vi "WSVCAP SHL Host TL RFFE Read.vi"(0 "Write Data In [DUT Ordered]":u8[][](array[numeric]) format="%02x", 7 "Socket Mask":u64=1 format="%016x", 11 "error in":errorcluster, 13 "Log (T)":bool=TRUE, 14 "FPGA":T1) -> (4 "Read Data Out":u8[][](array[numeric]) format="%.0x", 15 "error out":errorcluster)   [LabVIEW 2017]
uses:
  Type Defs/WSVCAP SHL FPGA Enum.ctl
  Type Defs/WSVCAP SHL Function Enum.ctl
panel:
  out "Status":u8[](array[numeric])
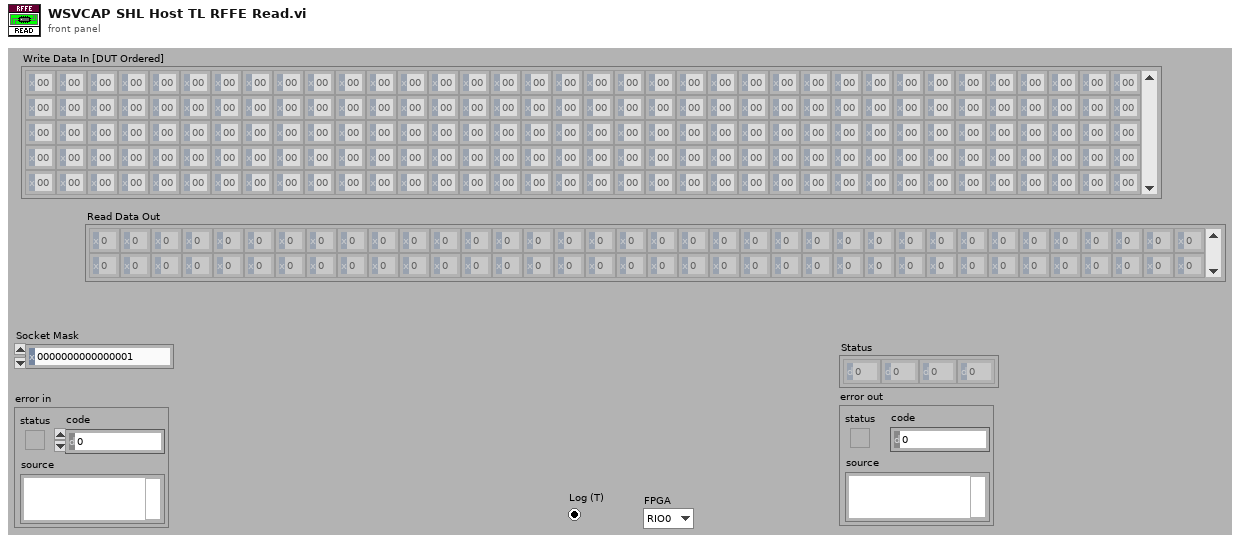
[diagram p1: front panel]
types:
  T1 = typedef "WSVCAP SHL FPGA Enum.ctl" = enum16{"RIO0", "RIO1"}
  T2 = typedef "WSVCAP SHL Function Enum.ctl" = enum16{"Initialize", "Configure I2C", "Configure RFFE", "Write I2C", "Read I2C", "Write RFFE", "Read RFFE", "Start RFFE Cycle", "Stop RFFE Cycle", "Get Status", "Close"}
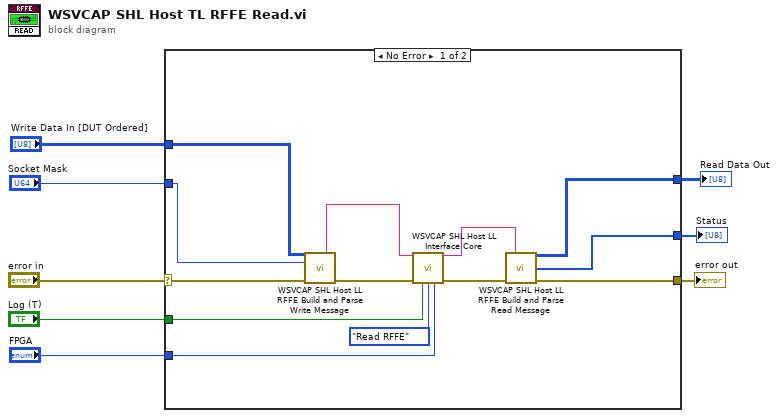
[diagram p0: block diagram]
diagram:
  n1 = case shown="No Error" "error in" {
    selector: "error in" -> [w14 w22]
    tunnel: [w18 w22] -> w8
    tunnel: "Socket Mask" -> [w12 _]
    tunnel: [w17 _] -> w5
    tunnel: [w16 _] -> w4
    tunnel: "Log (T)" -> [w15 _]
    tunnel: "Write Data In [DUT Ordered]" -> [w10 _]
    tunnel: "FPGA" -> [w9 _]
    frame No Error {
      n2 = call "WSVCAP SHL Host LL RFFE Build and Parse Write Message.vi"("Write Data In [DUT Ordered]"=w10, "Socket Mask [U64] In"=w12, "error in"=w14) -> ("Message Out"=w11:string, "error out"=w13:errorcluster)  [unwired: 6 in, 5 out]
      n3 = call "WSVCAP SHL Host LL Interface Core.vi"("Message In"=w11, "error in"=w13, "Log (T)"=w15, "Function"=WSVCAP_SHL_Function_Enum."Read RFFE", "FPGA"=w9) -> ("Message Out"=w19:string, "error out"=w20:errorcluster)  [unwired: 8 in, 1 out]
      n4 = call "WSVCAP SHL Host LL RFFE Build and Parse Read Message.vi"("Message In"=w19, "error in"=w20) -> ("Write Data Out"=w17:u8[][], "Status"=w16:u8[], "error out"=w18:errorcluster)  [unwired: 10 in, 1 out]
    }
    frame Error {
    }
  }
  "error out" <- w8
  "Read Data Out" <- w5
  "Status" <- w4
